vi "Untitled 1.vi"() -> ()   [LabVIEW 2020]
panel:
  out "Water level":dbl
  in  "Com Port":refnum<visa-resource-name>
  out "Tank":dbl(slide) scale=0.0..1000.0
  out "Pump Off":bool
  out "Pump On":bool
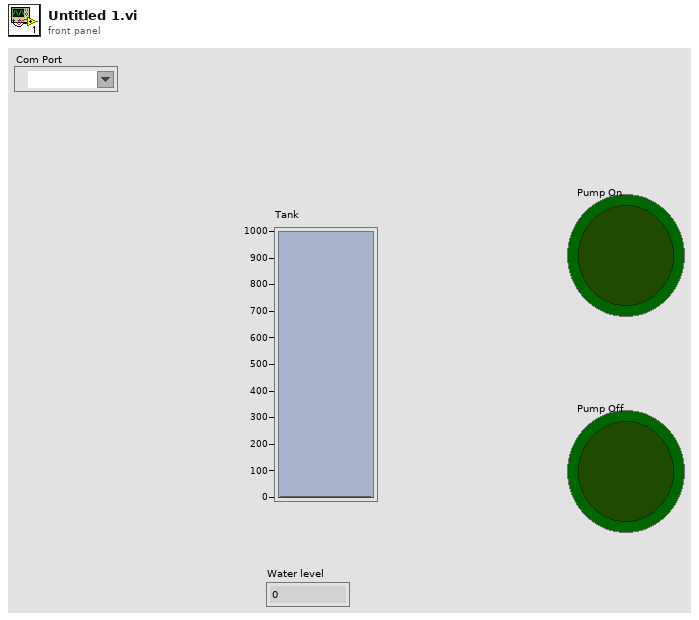
[diagram p1: front panel]
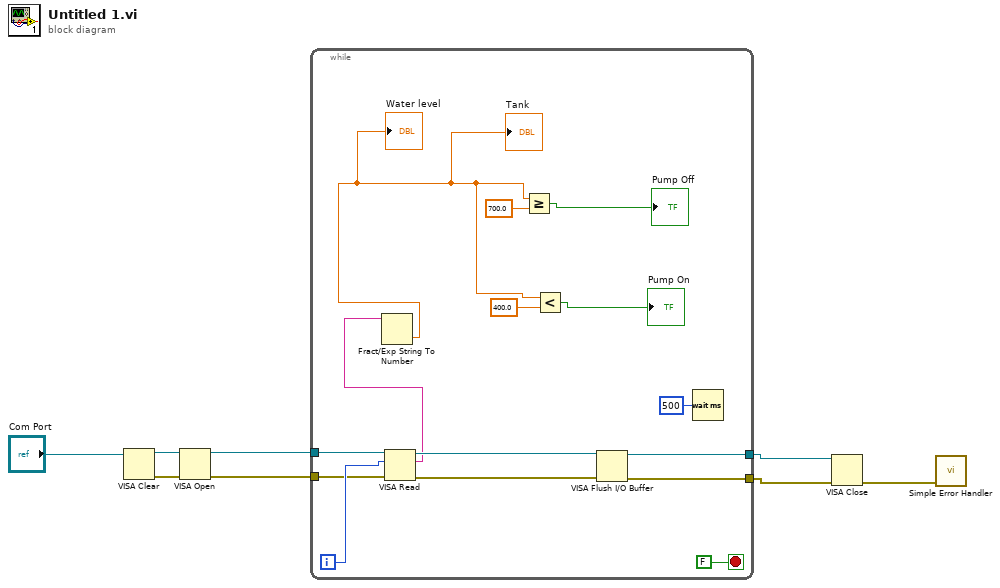
[diagram p0: block diagram]
diagram:
  n1 = VISA Clear(VISA resource name="Com Port") -> (VISA resource name out=w7:refnum<visa-resource-name>, error out=w8:errorcluster)  [unwired: 1 in]
  n2 = VISA Open(error in (no error)=w8, VISA resource name=w7) -> (VISA resource name=w3:refnum<visa-resource-name>, error out=w2:errorcluster)  [unwired: 3 in]
  n3 = while {
    tunnel: [w17] -> w5
    tunnel: [w16] -> w6
    tunnel: w3 -> [w15]
    tunnel: w2 -> [w14]
    i -> [w20]
    stop <- FALSE stop-if-true
    n4 = VISA Read(VISA resource name=w15, byte count=w20, error in (no error)=w14) -> (VISA resource name out=w19:refnum<visa-resource-name>, read buffer=w13:string, error out=w18:errorcluster)  [unwired: 1 out]
    n5 = Fract/Exp String To Number(string=w13) -> (number=w11:dbl)  [unwired: 3 in, 1 out]
    "Tank" <- w11
    "Water level" <- w11
    n6 = Greater Or Equal?(x=w11, y=700.0) -> (x >= y?=→"Pump Off":bool)
    n7 = Less?(x=w11, y=400.0) -> (x < y?=→"Pump On":bool)
    n8 = VISA Flush I/O Buffer(VISA resource name=w19, error in (no error)=w18) -> (VISA resource name out=w16:refnum<visa-resource-name>, error out=w17:errorcluster)  [unwired: 1 in]
    n9 = Wait (ms)(milliseconds to wait=u32 500) -> ()  [unwired: 1 out]
  }
  n10 = VISA Close(VISA resource name=w6, error in (no error)=w5) -> (error out=w4:errorcluster)
  n11 = call <vilib>:"Simple Error Handler.vi"("error in (no error)"=w4) -> ()  [unwired: 4 in, 5 out]
